vi "StopMotion.vi"(8 "error in (no error)":errorcluster, 11 "VXMx2 in":refnum<class "VXMx2.lvclass">) -> (0 "error out":errorcluster, 1 "All Positions, eng units":dbl[](array[numeric]), 3 "VXMx2 out":refnum<class "VXMx2.lvclass">)   [LabVIEW 2019, in "VXMx2.lvclass"]
uses:
  VXMx2.lvclass
  Support/MessageAPI/UIMessage.ctl
  VXMx2.lvclass/VXMx2.ctl
  SendMessage/SendMessage.lvclass
  <instrlib>/Velmex VXM/Velmex VXM.lvlib
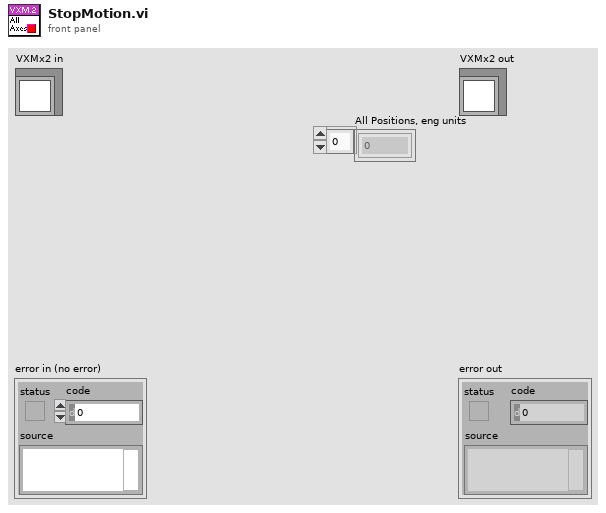
[diagram p1: front panel]
types:
  T1 = typedef "UIMessage.ctl" = cluster{"EventCode":i32, "Numeric":dbl, "String":string, "Variant":variant}
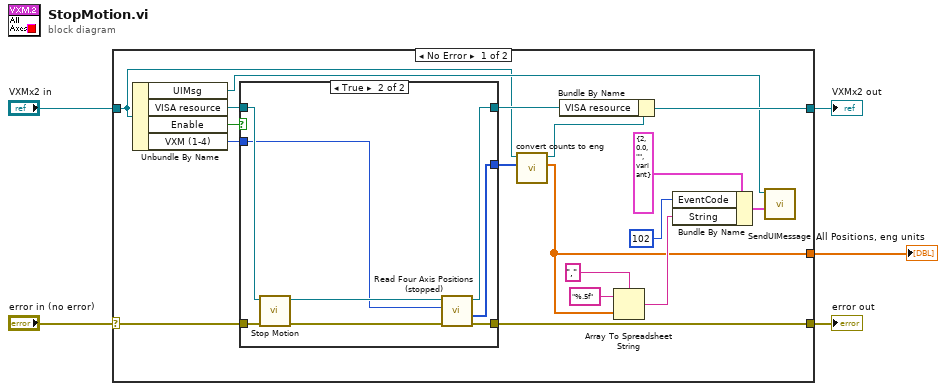
[diagram p0: block diagram]
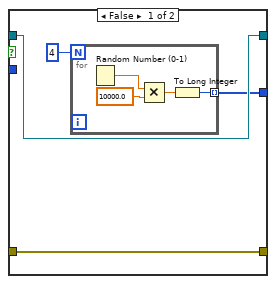
[diagram p2: hidden frame]
diagram:
  n1 = case shown="No Error" "error in (no error)" {
    selector: "error in (no error)" -> [w21 w41]
    tunnel: [w20 w41] -> w4
    tunnel: [w19 w40] -> w2
    tunnel: "VXMx2 in" -> [w12 w40]
    tunnel: [w6 _] -> w1
    frame No Error {
      n2 = Unbundle By Name(w12) -> ("UIMsg"=w17:refnum<class "SendMessage.lvclass">, "VISA resource"=w23:refnum<visa-resource-name>, "Enable"=w22:bool, "VXM (1-4)"=w7:i32)
      n3 = case shown="True" w22 {
        tunnel: w23 -> [w26 w39]
        tunnel: w21 -> [w27 w38]
        tunnel: [w27 w35] -> w20
        tunnel: [w26 w34] -> w18
        tunnel: [w24 w33] -> w13
        tunnel: w7 -> [_ w32]
        frame False {
          n4 = for {
            N: 4 -> [_]
            tunnel: [w28] -> w24 mode=indexing
            n5 = Random Number (0-1)() -> (number: 0 to 1=w31:dbl)
            n6 = Multiply(x=w31, y=10000.0) -> (x*y=w29:dbl)
            n7 = To Long Integer(number=w29) -> (32bit integer=w28:i32)
          }
        }
        frame True {
          n8 = call <instrlib>:"Stop Motion.vi"("error in (no error)"=w38, "VISA resource name"=w39) -> ("error out"=w37:errorcluster, "VISA resource out"=w36:refnum<visa-resource-name>)  [unwired: 8 in]
          n9 = call <instrlib>:"Read Four Axis Positions (stopped).vi"("error in (no error)"=w37, "VXM Model (1-4)"=w32, "VISA resource name"=w36) -> ("error out"=w35:errorcluster, "Positions, counts"=w33:i32[], "VISA resource out"=w34:refnum<visa-resource-name>)  [unwired: 6 in]
        }
      }
      n10 = call "convert counts to eng.vi"("All Positions, counts"=w13, "VXMx2 in"=w12) -> ("All Positions, eng units"=w6:dbl[], "VXMx2 out"=w11:refnum<class "VXMx2.lvclass">)  [unwired: 6 in, 2 out]
      n11 = Bundle By Name(cluster=w11, "VISA resource"=w18) -> (w19:refnum<class "VXMx2.lvclass">)
      n12 = Array To Spreadsheet String(delimiter (Tab)=",", array=w6, 3:"%.5f" ("format string")) -> (spreadsheet string=w9:string)
      n13 = Bundle By Name(cluster=T1 {"EventCode"=2, "Numeric"=0.0, "String"="", "Variant"=variant} ("UIMsg"), "EventCode"=102, "String"=w9) -> (w15:T1)
      n14 = call-dynamic "SendUIMessage.vi"("UIMsg"=w15, "SendMessage in"=w17) -> ()  [unwired: 8 in, 2 out]
    }
    frame Error {
    }
  }
  "error out" <- w4
  "VXMx2 out" <- w2
  "All Positions, eng units" <- w1
